vi "wa32 WriteFile with Timeout.vi"(7 "timeout [ms]":i32=3000, 8 "error in (no error)":errorcluster, 9 "write block size (10k)":i32=10000, 10 "data":u8[](array[numeric]), 11 "pipe handle":i32) -> (0 "error out":errorcluster, 2 "written":u32, 3 "pipe handle out":i32)   [LabVIEW 2020, in "GOLPI library.lvlib"]
doc: "Tries to write binary data to pipe with timeout. Note write block size must be smaller than pipe buffer size!"
uses:
  GOLPI library.lvlib
  <vilib>/Utility/error.llb/Error Cluster From Error Code.vi
  <vilib>/ErrorRing/Error Ring.xnode
panel:
  out "runtime written":u32
  out "write cycle":i32
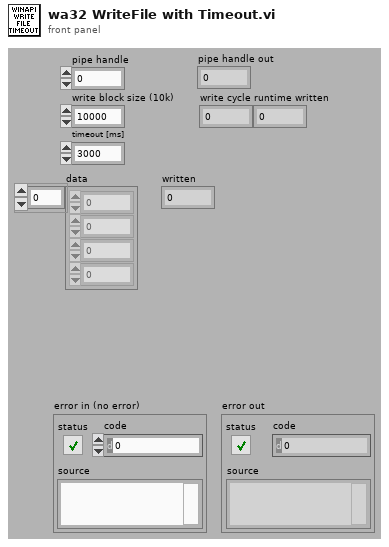
[diagram p1: front panel]
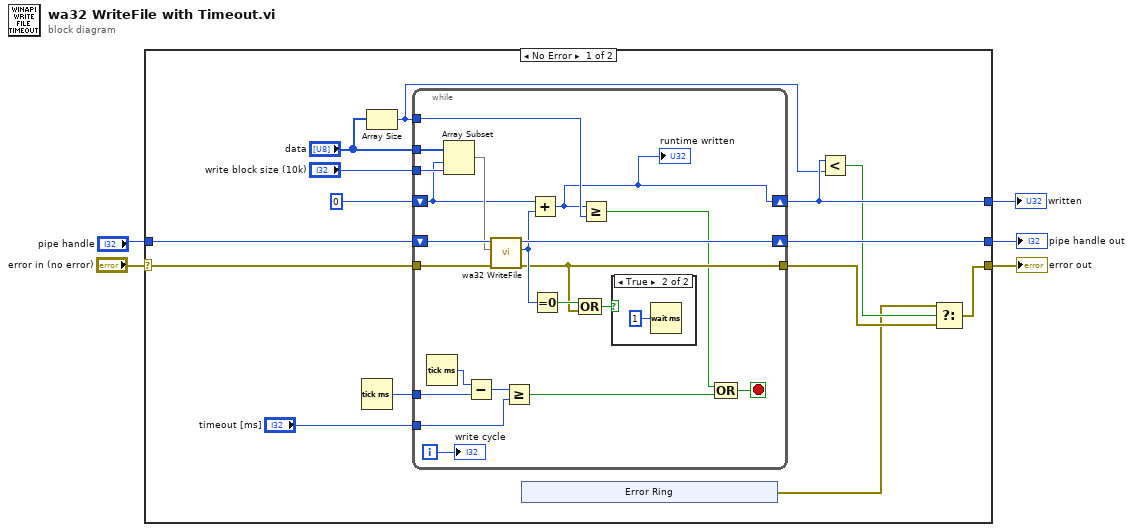
[diagram p0: block diagram]
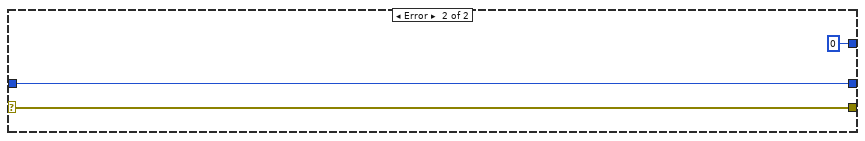
[diagram p3: hidden frame]
diagram:
  n1 = case shown="No Error" "error in (no error)" {
    selector: "error in (no error)" -> [w8 w49]
    tunnel: [w15 w47] -> w5
    tunnel: [w14 u32 0] -> w4
    tunnel: [w11 w49] -> w3
    tunnel: "pipe handle" -> [w7 w47]
    frame No Error {
      n2 = Tick Count (ms)() -> (millisecond timer value=w16:u32)
      n3 = Array Size(array="data") -> (size(s)=w13:i32)
      n4 = while {
        tunnel: w8 -> [w45]
        shift-right: [w43] -> w15
        shift-left: w7 -> [w44]
        tunnel: "data" -> [w42]
        tunnel: "write block size (10k)" -> [w41]
        shift-right: [w26] -> w14
        shift-left: 0 -> [w39]
        tunnel: w13 -> [w38]
        tunnel: [w35] -> w10
        tunnel: w16 -> [w32]
        tunnel: "timeout [ms]" -> [w29]
        i -> [w25]
        stop <- w27 stop-if-true
        n5 = Tick Count (ms)() -> (millisecond timer value=w33:u32)
        n6 = Array Subset(array=w42, index=w39, length=w41) -> (w40:u8[])
        n7 = Subtract(x=w33, y=w32) -> (x-y=w30:u32)
        n8 = call "wa32 WriteFile.vi"("error in"=w45, "data (empty)"=w40, "handle"=w44) -> ("error out"=w35:errorcluster, "written bytes"=w37:u32, "handle out"=w43:i32)  [unwired: 6 in]
        n9 = Greater Or Equal?(x=w30, y=w29) -> (x >= y?=w28:bool)
        n10 = Add(x=w39, y=w37) -> (x+y=w26:u32)
        "runtime written" <- w26
        n11 = Equal To 0?(x=w37) -> (x = 0?=w36:bool)
        n12 = Compound Arithmetic op=OR(w36, w35) -> (w34:bool)
        n13 = Greater Or Equal?(x=w26, y=w38) -> (x >= y?=w31:bool)
        n14 = case shown="True" w34 {
          frame False {
          }
          frame True {
            n15 = Wait (ms)(milliseconds to wait=u32 1) -> ()  [unwired: 1 out]
          }
        }
        n16 = Compound Arithmetic op=OR(w31, w28) -> (w27:bool)
        "write cycle" <- w25
      }
      n17 = xnode "Error Ring"() -> ("error out"=w9:errorcluster)
      n18 = Less?(x=w14, y=w13) -> (x < y?=w12:bool)
      n19 = Select(t=w9, s=w12, f=w10) -> (s? t:f=w11:errorcluster)
    }
    frame Error {
    }
  }
  "error out" <- w3
  "pipe handle out" <- w5
  "written" <- w4
